vi "Delegate.vi"(8 "error in (no error)":errorcluster, 10 "Action":T1={"Name"=enum."Drive Left", "Priority"=0, "Data"=variant}, 11 "Subsystems":refnum<queue>[](array[refnum])) -> (0 "error out":errorcluster, 3 "Delegate":refnum<queue>)   [LabVIEW 2015, in "Sprocket.lvlib"]
doc: "This VI demonstrates the most effort efficient method of leadership."
uses:
  lib/Sprocket.lvlib
  Action/Action.ctl
  Action/Action Name.ctl
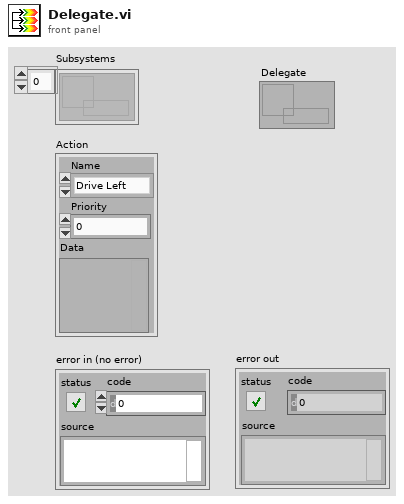
[diagram p1: front panel]
types:
  T1 = typedef "Sprocket.lvlib/Action.ctl" = cluster{"Name":T2, "Priority":i32, "Data":variant}
  T2 = typedef "Sprocket.lvlib/Action Name.ctl" = enum16{"No Action", "Drive Left", "Drive Right"}
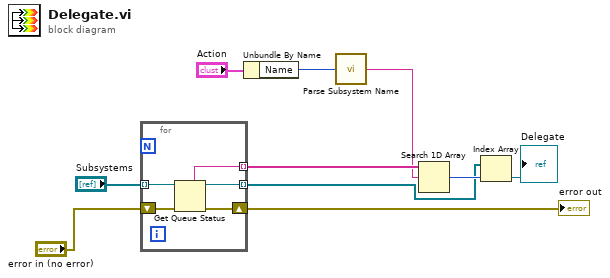
[diagram p0: block diagram]
diagram:
  n1 = for {
    tunnel: "Subsystems" -> [w15] mode=indexing
    shift-right: [w13] -> w8
    shift-left: "error in (no error)" -> [w14]
    tunnel: [w12] -> w5 mode=indexing
    tunnel: [w11] -> w2 mode=indexing
    n2 = Get Queue Status(queue=w15, error in (no error)=w14) -> (queue out=w11:refnum<queue>, queue name=w12:string, error out=w13:errorcluster)  [unwired: 1 in, 5 out]
  }
  "error out" <- w8
  n3 = Unbundle By Name("Action") -> ("Name"=w6:T2)
  n4 = call "Parse Subsystem Name.vi"("Action Enum"=w6) -> ("Subsystem Name"=w4:string)
  n5 = Search 1D Array(1D array=w5, element=w4) -> (index of element=w3:i32)  [unwired: 1 in]
  n6 = Index Array(array=w2, index=w3) -> (element=→"Delegate":refnum<queue>)
